vi "Main.vi"() -> ()   [LabVIEW 2020]
doc: "Main Program initialize config files, handles user inputs, image acquisition, object detection and image storing. User interface is handled in a state machine sending outputs."
uses:
  controls/State.ctl
  controls/Data.ctl
  <vilib>/userDefined/High Color/IMAQdx.ctl
  <vilib>/vision/Image Controls.llb/IMAQ Image.ctl
  b1a6e15a-21f6-4224-89c9-cebb1e441bce.vi
  4203ab90-da59-4329-829c-edbd02661f10.vi
  <extravilib>/ChannelInstances/Tag-bool/Read With Abort.vi
  <extravilib>/ChannelInstances/Tag-t'Data.ctl'/Read With Abort.vi
  <extravilib>/ChannelInstances/Tag-c(bool,bool)/Read With Abort.vi
  <extravilib>/ChannelInstances/Tag-c(bool,bool)/Write With Abort.vi
  <extravilib>/ChannelInstances/Tag-t'Data.ctl'/Write With Abort.vi
  <extravilib>/ChannelInstances/Tag-bool/Write With Abort.vi
  <extravilib>/ChannelInstances/Tag-c(bool,bool)/Instantiate.vi
  <extravilib>/ChannelInstances/Tag-t'Data.ctl'/Instantiate.vi
  <extravilib>/ChannelInstances/Tag-bool/Instantiate.vi
  <extravilib>/ChannelInstances/Tag-bool/EndpointRead.vi
  <extravilib>/ChannelInstances/Tag-t'Data.ctl'/EndpointRead.vi
  <extravilib>/ChannelInstances/Tag-c(bool,bool)/EndpointRead.vi
  <extravilib>/ChannelInstances/Tag-c(bool,bool)/Endpoint.vi
  <extravilib>/ChannelInstances/Tag-t'Data.ctl'/Endpoint.vi
  <extravilib>/ChannelInstances/Tag-bool/Endpoint.vi
  <extravilib>/ChannelInstances/Tag-bool.lvlib
  <extravilib>/ChannelInstances/Tag-t'Data.ctl'.lvlib
  <extravilib>/ChannelInstances/Tag-c(bool,bool).lvlib
panel:
  in  "Tab Control":T1(tab)
  in  "Sex":string="Station" caption="Sample Name"
  in  "Determiner":string="Station" caption="Sample Name"
  in  "Longitude":string="Station" caption="Sample Name"
  in  "Latitude":string="Station" caption="Sample Name"
  in  "Location":string="Station" caption="Sample Name"
  in  "Other notes":string caption="Sample Name"
  in  "Species Name":string="Test Sample" caption="Sample Name"
  in  "Station":string="Station" caption="Sample Name"
  in  "Collection date":string="24/06/2016" caption="Collection Date (DD/MM/YYYY)"
  out "Ready":bool
  in  "Operator":string="MRJ" caption="Sample Name"
  out "Active":bool
  in  "Start Image Capture":bool
  in  "Sample Name":string="#0000"
  in  "Stop Image Capture":bool
  out "Camera 2":bool
  out "Camear 1":bool
  out "Pump":bool
  out "Actuator":bool
  in  "Connect Systems":bool
  in  "Exit":bool
  in  "Empty and Refill":bool
  in  "Start System":bool
  in  "Empty System":bool
  out "Process buffer":T2(graph)
  out "Save buffer":T2(graph)
  in  "Close and Refill":bool
  in  "Manual Open":bool
  in  "Exposure Time":dbl=1000.0
  in  "Exposure":enum32{"Item 0", "Item 1", "Item 2", "Item 3"}(radio)=enum."Item 3"
  in  "Aperture":enum32{"Item 0", "Item 1", "Item 2", "Item 3"}(radio)
  in  "Flush Size":i32=100 min=0 max=1000
  in  "Dispense Duration":i32=200 min=20 max=200
  in  "Max large object threshold":i32=4 min=1
  in  "Change Crop":bool
  in  "DetectCrop":dbl=30.0 caption="Movement Detection size" format="%#_g %"
  in  "Sample size threshold":i32=500 min=1
  in  "New Sample timeout":i32=50 min=1
  out "Target framerate":i32=100
  in  "Light intensity":i32(slide)=100 min=1 max=100 scale=1.0..100.0 scale format="%.0f%"
  in  "Max Framerate":i32=100 min=1
  in  "Overload threshold":i32=50 min=1
  in  "Img Save Que Size":i32=100 caption="Image Save Queue Size" min=1
  in  "Img Proc Que Size":i32=200 caption="Image Processing Queue Size" min=1
  in  "Empty Cuvette":bool
  in  "Manual Close":bool
  out "Current Position":string
  in  "Position":bool
  in  "Pump Cycle":bool
  in  "Pump Bottom":bool
  in  "Pump Top":bool
  in  "Pump Terminate":bool
  in  "Override System":bool
  in  "Calibration Pictures":bool
  out "Framerate":i32 caption="Current Framerate"
  out "Camera 1":T3(plugin-control)
  out "Camera 2":T3(plugin-control)
  out "Camera 1 Binary":T3(plugin-control)
  out "Camera 2 Binary":T3(plugin-control)
  out "Camera 1 Detect":T3(plugin-control)
  out "Camera 2 Detect":T3(plugin-control)
  # "SRS Software - Version 1.5.3.2"
  # "Connections"
  # "Camera/Lens settings"
  # "Dispenser settings"
  # "Detection settings"
  # "Image capture settings"
  # "Buffer settings"
  # "Hatch control"
  # "Pump"
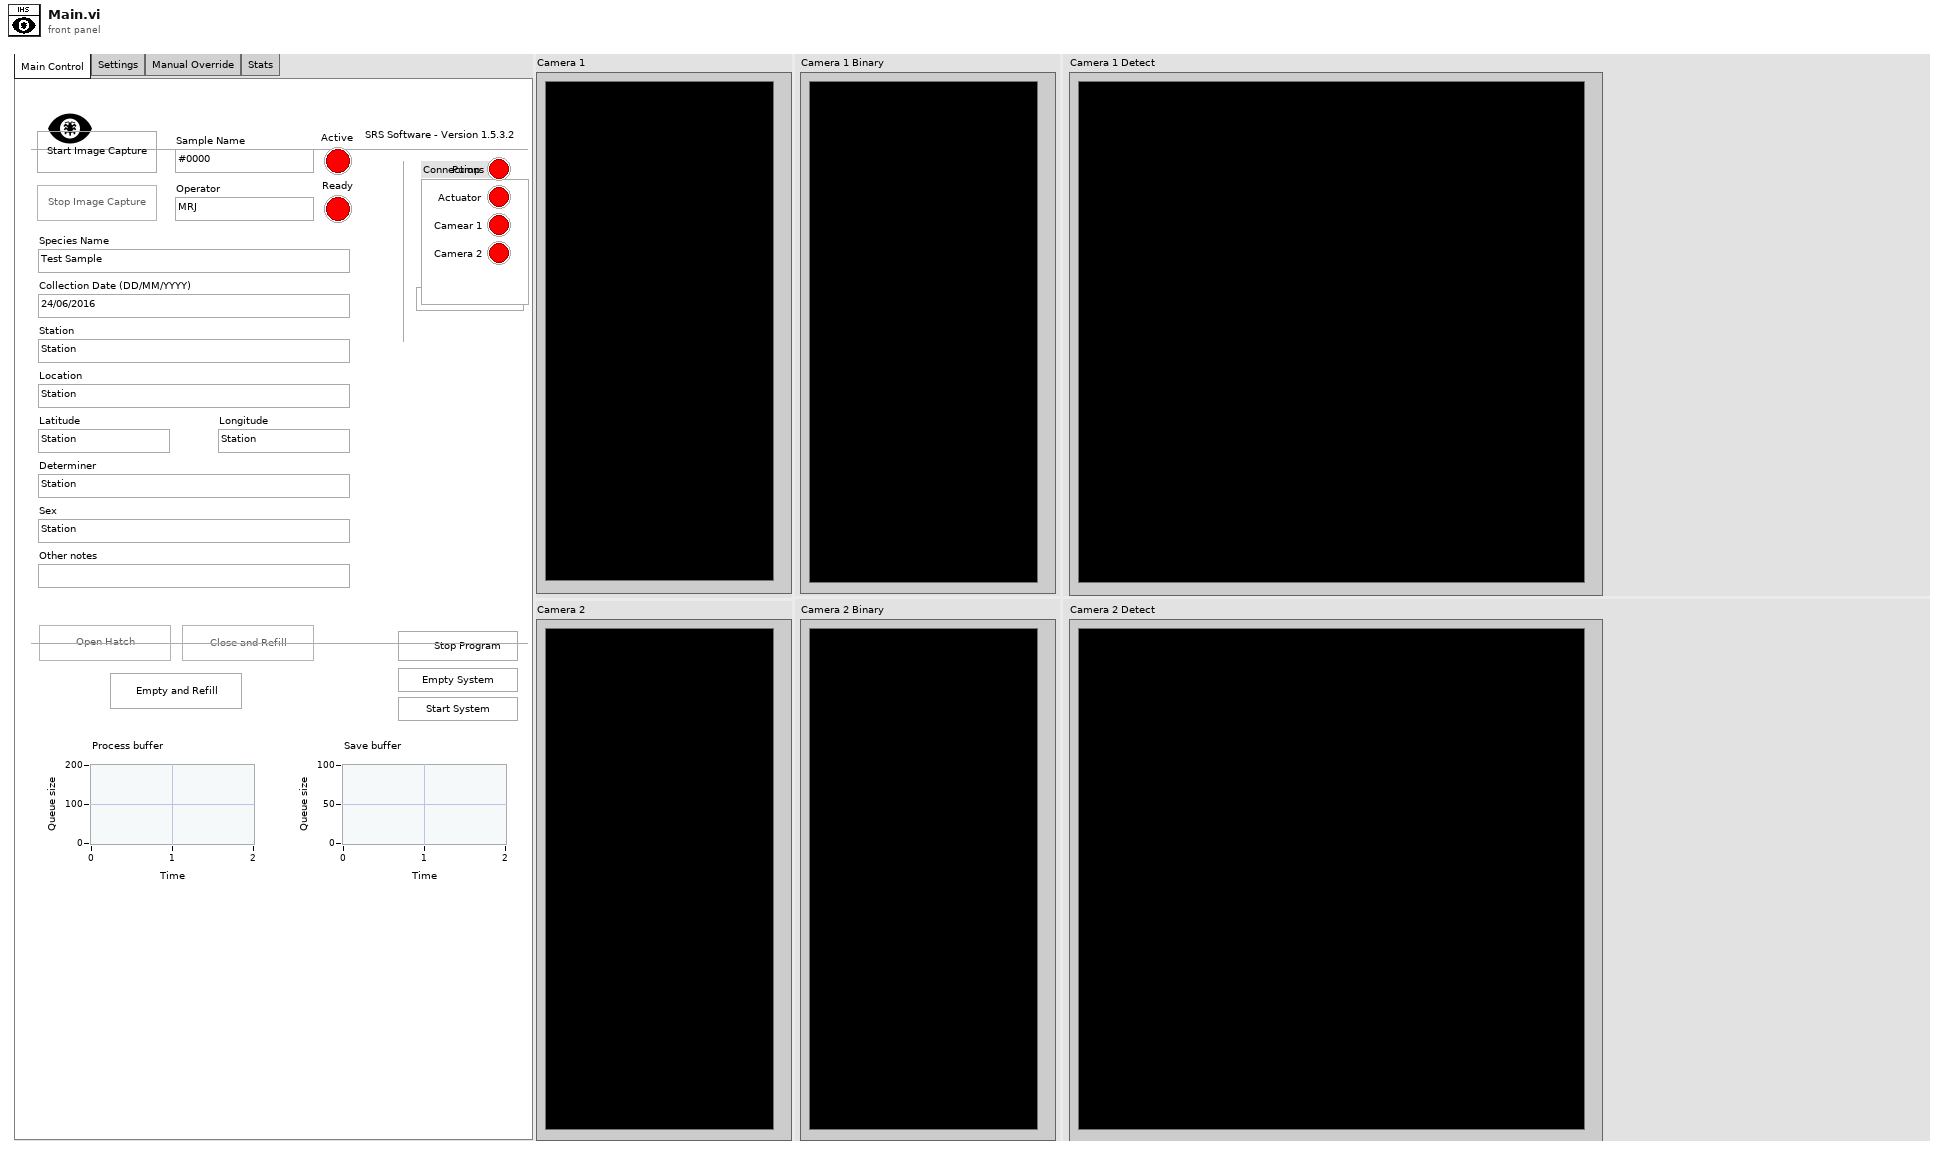
[diagram p1: front panel]
types:
  T1 = enum32{"Main Control", "Settings", "Manual Override", "Stats"}
  T2 = cluster{"# elements in queue":i32, "# elements in queue":i32}
  T3 = typedef "IMAQ Image.ctl" = refnum<image>
  T4 = typedef "Data.ctl" = cluster{"L16 Linear Actuator":refnum<visa-resource-name>, "XE 1000 Pump":refnum<visa-resource-name>, "Camera1":T5, "Camera2":T5, "Img_Capt":bool, "Actuator":bool, "Pump":bool, "Cam 1":bool, "Cam 2":bool, "Empty_Refill":bool, "Crop":bool, "Light intensity":i32, "Exposure Time":dbl, "Sample Name":string, "Operator":string, "Calibration 1":path, "Calibration 2":path, "Framerate":i32, "Timeout Sample":i32, "Collection date":string, "Sample size threshold":i32, "Empty start":u32, "Command":string, "Station":string, "Species Name":string, "Other Notes":string, "Aperture":enum32{"Item 0", "Item 1", "Item 2", "Item 3"}, "Image Process Queue Size":i32, "Image Save Queue Size":i32, "Overload threshold":i32, "Max Framerate":i32, "Rectangle 1":T6, "Rectangle 2":T6, "Detection Region %":dbl, "Detect 1":path, "Detect 2":path, "Max large object threshold":i32, "Open(T)/Close(F)":bool, "Img_Capt Begin":bool, "Dispense Speed":i32, "Flush Size":i32, "Location":string, "Latitude":string, "Longitude":string, "Determiner":string, "Sex":string, "Camera1_Img":T3, "Camera2_Img":T3, "Img1_Orig_Disp":T3, "Img2_Orig_Disp":T3, "Img1_Orig_RGB":T3, "Img2_Orig_RGB":T3, "Blue_Plane_Extract":T3, "Subtracted_Plane":T3, "Img1_Binary":T3, "Img2_Binary":T3, "Crop_Mask":T3, "Img1_Save":T3, "Img2_Save":T3, "Img1_Cali_Full":T3, "Img2_Cali_Full":T3, "Img1_Cali_Detect":T3, "Img2_Cali_Detect":T3, "Cam 1 queue":refnum<queue>, "Cam 1 - save queue":refnum<queue>, "Cam 2 queue":refnum<queue>, "Cam 2 - save queue":refnum<queue>}
  T5 = typedef "IMAQdx.ctl" = refnum<k21>
  T6 = typedef "IMAQ Rectangle" = cluster{"Left":i32, "Top":i32, "Right":i32, "Bottom":i32, "Rotation":dbl}
  T7 = typedef "State.ctl" = enum16{"Initialize", "Wait for Event", "Position", "Valve Signal", "Extra Flush", "Valve Cycle", "Valve Open", "Valve Close", "Pump Command", "Pump Cycle", "Empty System", "Start System", "Connect Systems", "Start Image Capture", "Stop Image Capture", "Calibration Pictures", "Close and Refill", "Empty and Refill", "Change Light Intensity", "Reconnect", "Exit"}
  T8 = enum8{"Enabled", "Disabled", "Disabled and Grayed Out"}
  T9 = cluster{"# elements in queue":i32, "# elements in queue":i32}[]
  T10 = typedef "Tag-t'Data.ctl'.lvlib/))Channel.ctl" = refnum<queue>
  T11 = typedef "Tag-bool.lvlib/))Channel.ctl" = refnum<queue>
  T12 = typedef "Tag-c(bool,bool).lvlib/))Channel.ctl" = refnum<queue>
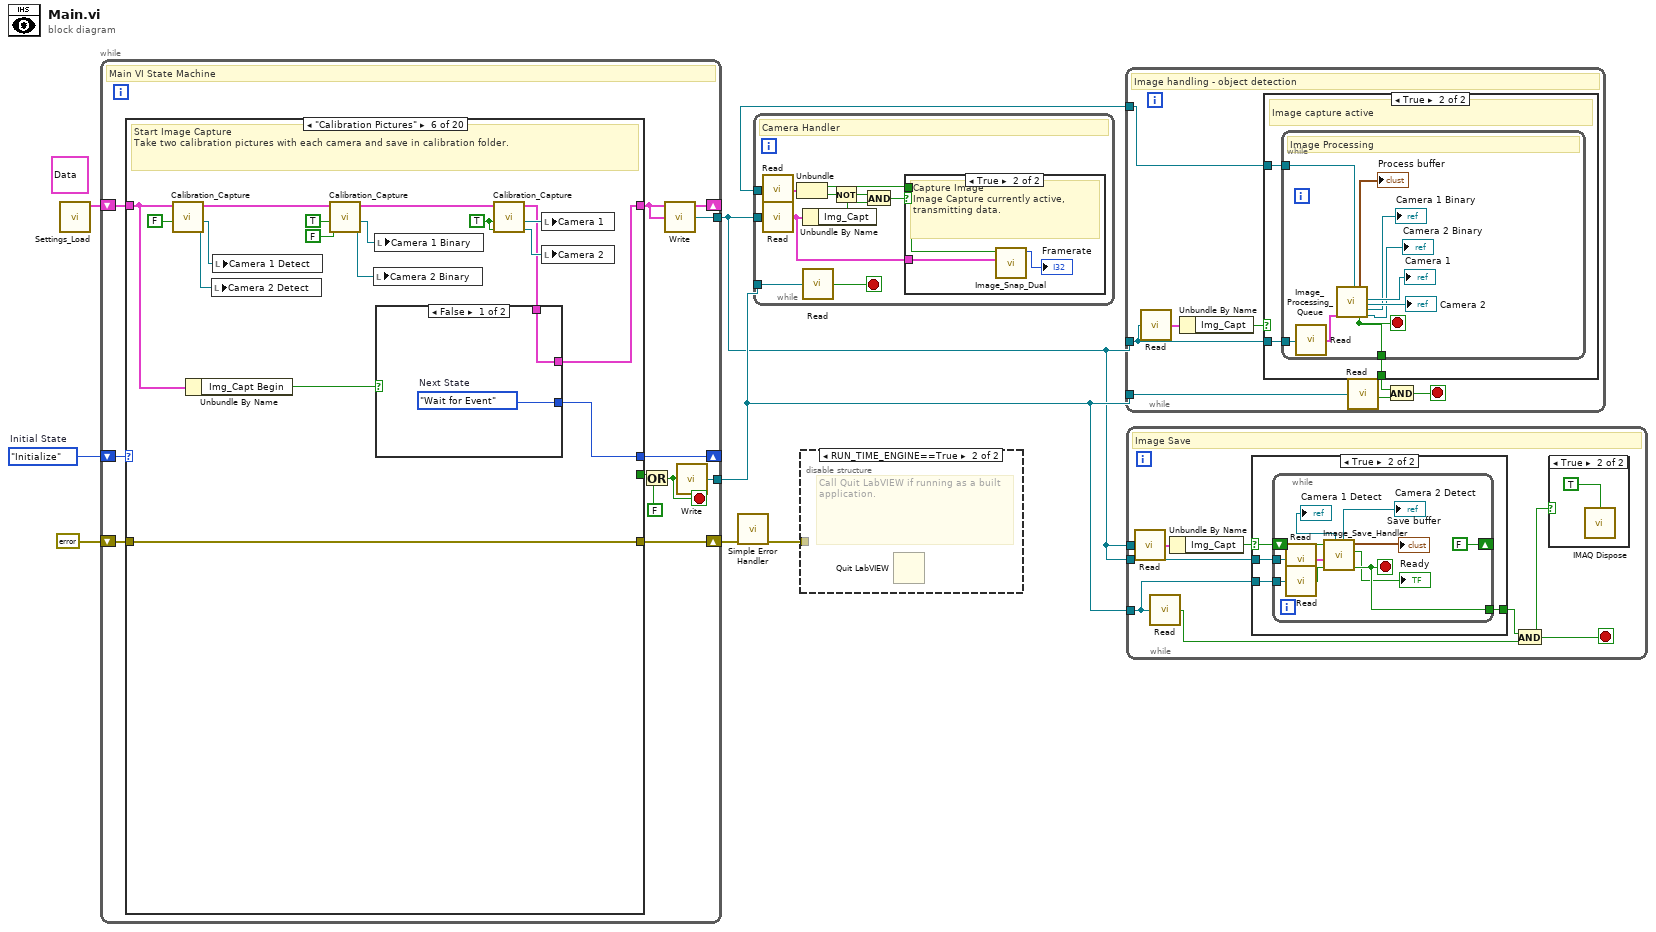
[diagram p0: block diagram]
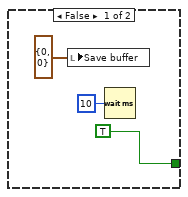
[diagram p3: hidden frame]
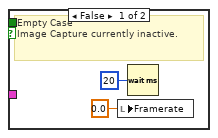
[diagram p4: hidden frame]
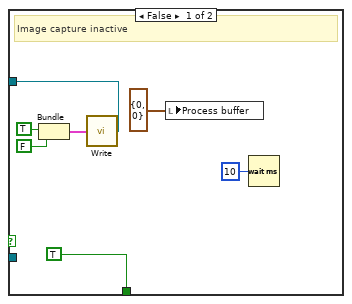
[diagram p5: hidden frame]
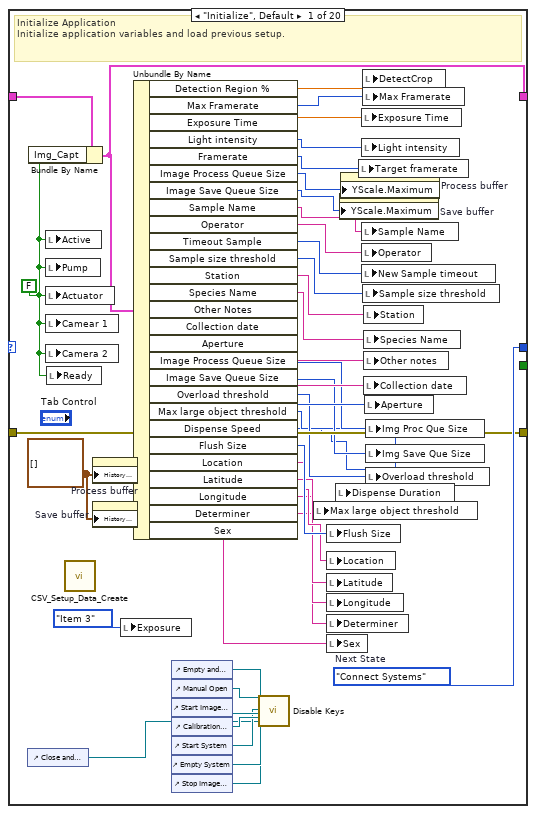
[diagram p7: hidden frame]
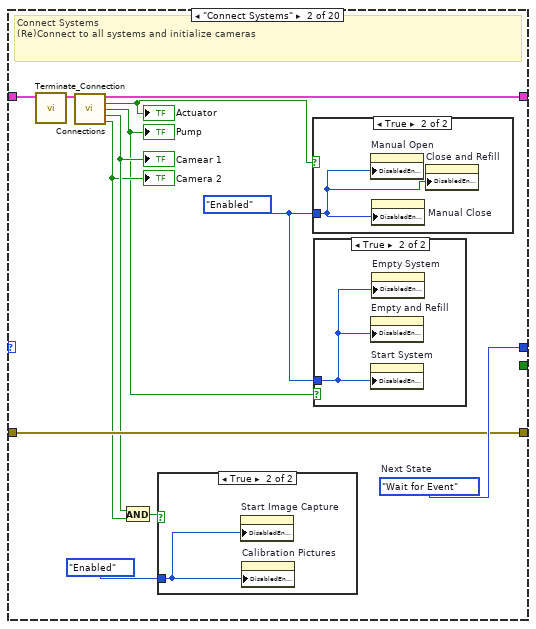
[diagram p8: hidden frame]
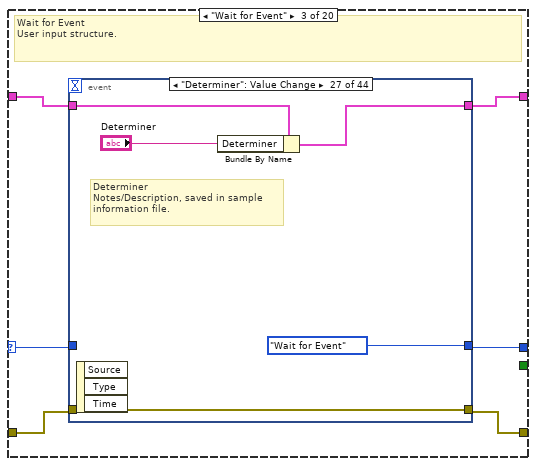
[diagram p12: hidden frame]
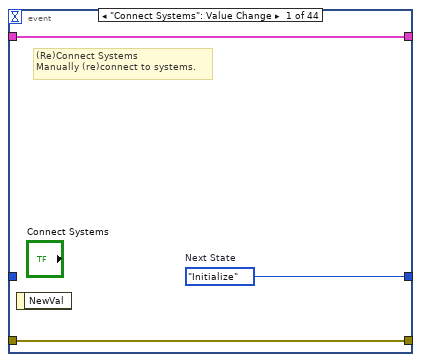
[diagram p13: hidden frame]
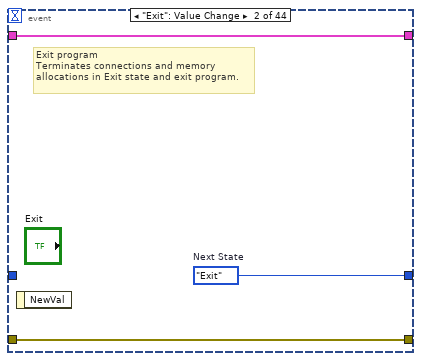
[diagram p14: hidden frame]
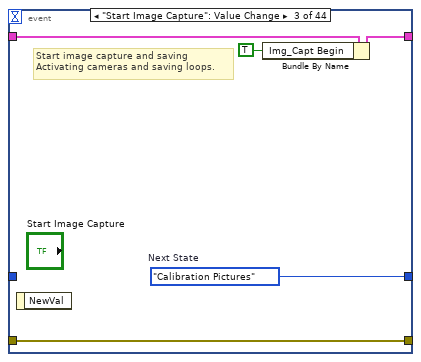
[diagram p15: hidden frame]
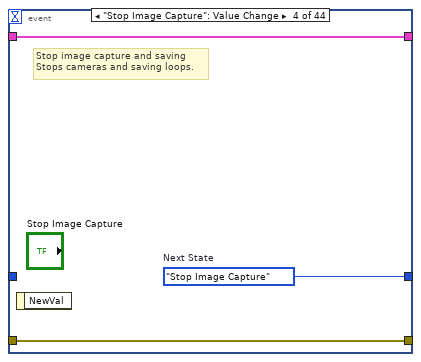
[diagram p16: hidden frame]
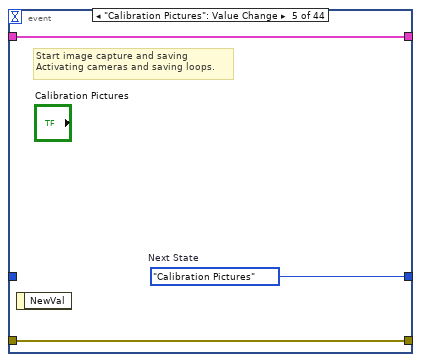
[diagram p17: hidden frame]
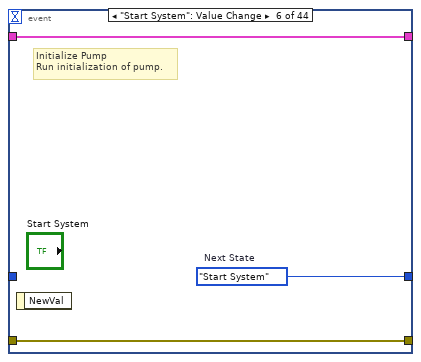
[diagram p18: hidden frame]
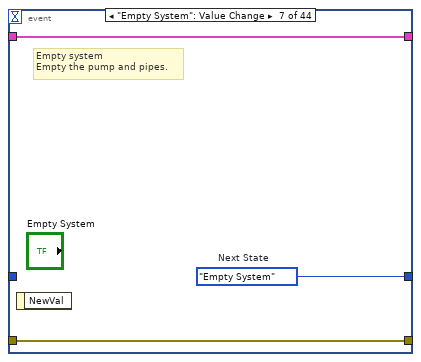
[diagram p19: hidden frame]
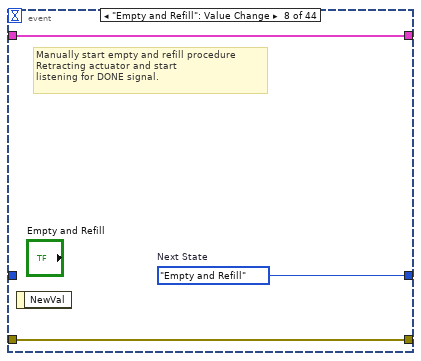
[diagram p20: hidden frame]
diagram:
  (unwired) T4 {"L16 Linear Actuator"="", "XE 1000 Pump"="", "Camera1"="", "Camera2"="", "Img_Capt"=FALSE, "Actuator"=FALSE, "Pump"=FALSE, "Cam 1"=FALSE, "Cam 2"=FALSE, "Empty_Refill"=FALSE, "Crop"=FALSE, "Light intensity"=100, "Exposure Time"=1000.0, "Sample Name"="Test Sample", "Operator"="MRJ", "Calibration 1"=path "C:/Users/au540322/Desktop/IHS_Project/images/Debris/Debris_0/Debris_0_2019_06_01-23-32-49-686.PNG", "Calibration 2"=path "C:/Users/au540322/Desktop/IHS_Project/images/Debris/Debris_0/Debris_0_2019_06_01-23-32-49-686.PNG", "Framerate"=100, "Timeout Sample"=200, "Collection date"="", "Sample size threshold"=500, "Empty start"=1, "Command"="", "Station"="", "Species Name"="", "Other Notes"="", "Aperture"=enum."Item 0", "Image Process Queue Size"=500, "Image Save Queue Size"=500, "Overload threshold"=500, "Max Framerate"=100, "Rectangle 1"={"Left"=0, "Top"=0, "Right"=0, "Bottom"=0, "Rotation"=0.0}, "Rectangle 2"={"Left"=0, "Top"=0, "Right"=0, "Bottom"=0, "Rotation"=0.0}, "Detection Region %"=0.0, "Detect 1"=path "C:/Users/au540322/Desktop/IHS_Project/images/Debris/Debris_0/Debris_0_2019_06_01-23-32-49-686.PNG", "Detect 2"=path "C:/Users/au540322/Desktop/IHS_Project/images/Debris/Debris_0/Debris_0_2019_06_01-23-32-49-686.PNG", "Max large object threshold"=0, "Open(T)/Close(F)"=FALSE, "Img_Capt Begin"=FALSE, "Dispense Speed"=100, "Flush Size"=100, "Location"="Station", "Latitude"="Station", "Longitude"="Station", "Determiner"="Station", "Sex"="Station", "Camera1_Img"=refnum, "Camera2_Img"=refnum, "Img1_Orig_Disp"=refnum, "Img2_Orig_Disp"=refnum, "Img1_Orig_RGB"=refnum, "Img2_Orig_RGB"=refnum, "Blue_Plane_Extract"=refnum, "Subtracted_Plane"=refnum, "Img1_Binary"=refnum, "Img2_Binary"=refnum, "Crop_Mask"=refnum, "Img1_Save"=refnum, "Img2_Save"=refnum, "Img1_Cali_Full"=refnum, "Img2_Cali_Full"=refnum, "Img1_Cali_Detect"=refnum, "Img2_Cali_Detect"=refnum, "Cam 1 queue"=refnum, "Cam 1 - save queue"=refnum, "Cam 2 queue"=refnum, "Cam 2 - save queue"=refnum} ("Data")
  w8 = State."Initialize"  # Initial State
  n1 = call "Settings_Load.vi"() -> ("value"=w4:T4)  [unwired: 10 in, 1 out]
  n2 = while {
    shift-right: [w18] -> _
    shift-left: w8 -> [w19]
    shift-right: [w16] -> _
    shift-left: w4 -> [w17]
    shift-right: [w13] -> w6
    shift-left: errorcluster {"status"=FALSE, "code"=0, "source"=""} ("error constant") -> [w15]
    tunnel: [w10] -> w3
    tunnel: [w11] -> w2
    stop <- w14 stop-if-true
    # "Main VI State Machine"
    n3 = case shown="\"Calibration Pictures\"" w19 {
      selector: w19 -> [_ _ w77 _ _ _ _ _ _ _ _ _ _ _ _ _ _ _ _ _]
      tunnel: [w61 w73 w82 w311 w329 w347 w376 w401 w407 w424 w441 w449 w462 w480 w490 w520 w542 w560 w563 w576] -> w18
      tunnel: [_ _ _ _ _ _ _ _ _ _ _ _ _ _ _ _ _ _ _ w575] -> w12
      tunnel: w17 -> [w53 w70 w81 w312 w325 w340 w370 w395 w411 w428 w433 w447 w460 w479 w484 w519 w532 w544 w567 w569]
      tunnel: [w59 w71 w80 w313 w327 w339 w375 w400 w402 w428 w434 w444 w459 w479 w483 w519 w531 w543 w567 w572] -> w16
      tunnel: w15 -> [w60 w72 w79 w314 w328 w346 w365 w390 w410 w425 w439 w452 w464 w475 w487 w516 w539 w557 w566 w574]
      tunnel: [w60 w72 w78 w314 w328 w346 w359 w383 w410 w418 w438 w450 w453 w474 w486 w513 w538 w548 w564 w568] -> w13
      frame "Initialize", Default {
        w52 = T9 [] ("History Data")
        w51 = FALSE ("Pump")
        w61 = State."Connect Systems"  # Next State
        # "Initialize Application\nInitialize application variables and load previous setup."
        n4 = control-ref of="Close and Refill"() -> (w33:refnum<vi>)
        n5 = Bundle By Name(cluster=w53, "Img_Capt"=w51) -> (w59:T4)
        n6 = local write "Active"(w51) -> ()
        n7 = local write "Pump"(w51) -> ()
        n8 = local write "Actuator"(w51) -> ()
        n9 = local write "Camear 1"(w51) -> ()
        n10 = local write "Camera 2"(w51) -> ()
        n11 = local write "Ready"(w51) -> ()
        n12 = call "CSV_Setup_Data_Create.vi"() -> ()  [unwired: 11 in, 1 out]
        n13 = property on="Process buffer" class="WFChart (strict)"("History Data"=w52) -> ()  [unwired: 2 in, 2 out]
        n14 = property on="Save buffer" class="WFChart (strict)"("History Data"=w52) -> ()  [unwired: 2 in, 2 out]
        n15 = local write "Exposure"(enum32{"Item 0", "Item 1", "Item 2", "Item 3"}."Item 3" ("Exposure")) -> ()
        n16 = Unbundle By Name(w59) -> ("Detection Region %"=w30:dbl, "Max Framerate"=w31:i32, "Exposure Time"=w58:dbl, "Light intensity"=w57:i32, "Framerate"=w56:i32, "Image Process Queue Size"=w29:i32, "Image Save Queue Size"=w28:i32, "Sample Name"=w55:string, "Operator"=w54:string, "Timeout Sample"=w50:i32, "Sample size threshold"=w49:i32, "Station"=w48:string, "Species Name"=w47:string, "Other Notes"=w46:string, "Collection date"=w45:string, "Aperture"=w44:enum32{"Item 0", "Item 1", "Item 2", "Item 3"}, "Image Process Queue Size"=w43:i32, "Image Save Queue Size"=w42:i32, "Overload threshold"=w41:i32, "Max large object threshold"=w27:i32, "Dispense Speed"=w25:i32, "Flush Size"=w26:i32, "Location"=w24:string, "Latitude"=w23:string, "Longitude"=w22:string, "Determiner"=w21:string, "Sex"=w20:string)
        n17 = control-ref of="Empty and Refill"() -> (w40:refnum<vi>)
        n18 = control-ref of="Manual Open"() -> (w39:refnum<vi>)
        n19 = control-ref of="Start Image Capture"() -> (w37:refnum<vi>)
        n20 = control-ref of="Calibration Pictures"() -> (w38:refnum<vi>)
        n21 = control-ref of="Start System"() -> (w36:refnum<vi>)
        n22 = control-ref of="Empty System"() -> (w35:refnum<vi>)
        n23 = control-ref of="Stop Image Capture"() -> (w34:refnum<vi>)
        n24 = call "Disable Keys.vi"("Boolean in"=w39, "Bool Refnum 6"=w40, "Bool Refnum 4"=w34, "Bool Refnum 7"=w36, "Bool Refnum 9"=w37, "Bool Refnum 2"=w38, "Bool Refnum 8"=w33, "Bool Refnum 3"=w35) -> ()  [unwired: 20 in]
        n25 = local write "Max large object threshold"(w27) -> ()
        n26 = local write "Flush Size"(w26) -> ()
        n27 = local write "Location"(w24) -> ()
        n28 = local write "Latitude"(w23) -> ()
        n29 = local write "Longitude"(w22) -> ()
        n30 = local write "Determiner"(w21) -> ()
        n31 = local write "Sex"(w20) -> ()
        n32 = local write "Dispense Duration"(w25) -> ()
        n33 = property on="Save buffer" class="WFChart (strict)"("YScale.Maximum"=w28) -> ()  [unwired: 2 in, 2 out]
        n34 = property on="Process buffer" class="WFChart (strict)"("YScale.Maximum"=w29) -> ()  [unwired: 2 in, 2 out]
        n35 = local write "Target framerate"(w56) -> ()
        n36 = local write "Exposure Time"(w58) -> ()
        n37 = local write "Light intensity"(w57) -> ()
        n38 = local write "Sample Name"(w55) -> ()
        n39 = local write "Operator"(w54) -> ()
        n40 = local write "New Sample timeout"(w50) -> ()
        n41 = local write "DetectCrop"(w30) -> ()
        n42 = local write "Max Framerate"(w31) -> ()
        n43 = local write "Sample size threshold"(w49) -> ()
        n44 = local write "Station"(w48) -> ()
        n45 = local write "Species Name"(w47) -> ()
        n46 = local write "Other notes"(w46) -> ()
        n47 = local write "Collection date"(w45) -> ()
        n48 = local write "Aperture"(w44) -> ()
        n49 = local write "Img Proc Que Size"(w43) -> ()
        n50 = local write "Img Save Que Size"(w42) -> ()
        n51 = local write "Overload threshold"(w41) -> ()
      }
      frame "Connect Systems" {
        w62 = T8."Enabled" ("Disabled")
        w73 = State."Wait for Event"  # Next State
        # "Connect Systems\n(Re)Connect to all systems and initialize cameras"
        n52 = call "Terminate_Connection.vi"("Data"=w70) -> ("Data out"=w69:T4)  [unwired: 9 in, 1 out]
        n53 = call "Connections.vi"("input cluster"=w69) -> ("output cluster"=w71:T4, "Linear Actuator"=w68:bool, "Pump"=w64:bool, "Camear 1"=w66:bool, "Camera 2"=w65:bool)  [unwired: 10 in]
        "Pump" <- w64
        "Actuator" <- w68
        "Camera 2" <- w65
        "Camear 1" <- w66
        n54 = And(x=w66, y=w65) -> (x .and. y?=w67:bool)
        n55 = case shown="True" w67 {
          tunnel: T8."Enabled" ("Disabled") -> [_ w75]
          frame False {
          }
          frame True {
            n56 = property on="Start Image Capture" class="Bool"("DisabledEnum"=w75) -> ()  [unwired: 2 in, 2 out]
            n57 = property on="Calibration Pictures" class="Bool"("DisabledEnum"=w75) -> ()  [unwired: 2 in, 2 out]
          }
        }
        n58 = case shown="True" w68 {
          tunnel: w62 -> [_ w76]
          frame False {
          }
          frame True {
            n59 = property on="Manual Open" class="Bool"("DisabledEnum"=w76) -> ()  [unwired: 2 in, 2 out]
            n60 = property on="Manual Close" class="Bool"("DisabledEnum"=w76) -> ()  [unwired: 2 in, 2 out]
            n61 = property on="Close and Refill" class="Bool"("DisabledEnum"=w76) -> ()  [unwired: 2 in, 2 out]
          }
        }
        n62 = case shown="True" w64 {
          tunnel: w62 -> [_ w74]
          frame False {
          }
          frame True {
            n63 = property on="Empty and Refill" class="Bool"("DisabledEnum"=w74) -> ()  [unwired: 2 in, 2 out]
            n64 = property on="Start System" class="Bool"("DisabledEnum"=w74) -> ()  [unwired: 2 in, 2 out]
            n65 = property on="Empty System" class="Bool"("DisabledEnum"=w74) -> ()  [unwired: 2 in, 2 out]
          }
        }
      }
      frame "Wait for Event" {
        # "Wait for Event\nUser input structure."
        n66 = event shown="[26] \"Determiner\": Value Change" {
          selector: _ -> [_ _ _ _ _ _ _ _ _ _ _ _ _ _ _ _ _ _ _ _ _ _ _ _ _ _ _ _ _ _ _ _ _ _ _ _ _ _ _ _ _ _ _ _]
          dyn-events: _ -> [_ _ _ _ _ _ _ _ _ _ _ _ _ _ _ _ _ _ _ _ _ _ _ _ _ _ _ _ _ _ _ _ _ _ _ _ _ _ _ _ _ _ _ _]
          timeout: _ -> [_ _ _ _ _ _ _ _ _ _ _ _ _ _ _ _ _ _ _ _ _ _ _ _ _ _ _ _ _ _ _ _ _ _ _ _ _ _ _ _ _ _ _ _]
          tunnel: [w85 w88 w93 w96 w99 w102 w105 w108 w111 w122 w125 w128 w131 w134 w137 w142 w147 w152 w153 w158 State."Wait for Event" ("Next State") State."Wait for Event" ("Next State") State."Wait for Event" ("Next State") State."Wait for Event" ("Next State") State."Wait for Event" ("Next State") State."Wait for Event" ("Next State") State."Wait for Event" ("Next State") State."Wait for Event" ("Next State") State."Wait for Event" ("Next State") State."Wait for Event" ("Next State") State."Wait for Event" ("Next State") State."Wait for Event" ("Next State") w245 w250 w255 w260 w265 w277 State."Change Light Intensity" ("Next State") w286 w291 State."Change Light Intensity" ("Next State") State."Wait for Event" ("Next State") w308] -> w82
          tunnel: w81 -> [w83 w87 w91 w94 w97 w100 w103 w106 w109 w120 w123 w126 w129 w132 w135 w139 w144 w149 w156 w159 w164 w168 w174 w179 w184 w189 w194 w199 w204 w211 w216 w239 w246 w251 w256 w261 w266 w270 w283 w288 w293 w298 w303 w306]
          tunnel: [w83 w87 w90 w94 w97 w100 w103 w106 w109 w120 w123 w126 w129 w132 w135 w138 w143 w148 w155 w160 w165 w169 w175 w180 w185 w190 w195 w200 w205 w208 w224 w240 w247 w252 w257 w262 w267 w278 w282 w287 w292 w297 w302 w305] -> w80
          tunnel: w79 -> [w84 w86 w92 w95 w98 w101 w104 w107 w110 w121 w124 w127 w130 w133 w136 w141 w146 w151 w157 w162 w167 w172 w177 w182 w187 w192 w197 w202 w207 w213 w226 w243 w248 w253 w258 w263 w268 w279 w284 w289 w294 w299 w304 w307]
          tunnel: [w84 w86 w92 w95 w98 w101 w104 w107 w110 w121 w124 w127 w130 w133 w136 w141 w146 w151 w157 w162 w167 w172 w177 w182 w187 w192 w197 w202 w207 w213 w226 w243 w248 w253 w258 w263 w268 w279 w284 w289 w294 w299 w304 w307] -> w78
          tunnel: w77 -> [_ _ _ _ _ _ _ _ _ _ _ _ _ _ _ _ _ _ _ _ _ _ _ _ _ _ _ _ _ _ _ _ _ _ _ _ _ _ _ _ _ _ _ _]
          event "Connect Systems": Value Change {
            w85 = State."Initialize"  # Next State
            # "(Re)Connect Systems\nManually (re)connect to systems."
            n67 = event-data() -> ()  [unwired: 1 in, 1 out]
          }
          event "Exit": Value Change {
            w88 = State."Exit"  # Next State
            # "Exit program\nTerminates connections and memory\nallocations in Exit state and exit program."
            n68 = event-data() -> ()  [unwired: 1 in, 1 out]
          }
          event "Start Image Capture": Value Change {
            w93 = State."Calibration Pictures"  # Next State
            # "Start image capture and saving\nActivating cameras and saving loops."
            n69 = event-data() -> ()  [unwired: 1 in, 1 out]
            n70 = Bundle By Name(cluster=w91, "Img_Capt Begin"=TRUE) -> (w90:T4)
          }
          event "Stop Image Capture": Value Change {
            w96 = State."Stop Image Capture"  # Next State
            # "Stop image capture and saving\nStops cameras and saving loops."
            n71 = event-data() -> ()  [unwired: 1 in, 1 out]
          }
          event "Calibration Pictures": Value Change {
            w99 = State."Calibration Pictures"  # Next State
            # "Start image capture and saving\nActivating cameras and saving loops."
            n72 = event-data() -> ()  [unwired: 1 in, 1 out]
          }
          event "Start System": Value Change {
            w102 = State."Start System"  # Next State
            # "Initialize Pump\nRun initialization of pump."
            n73 = event-data() -> ()  [unwired: 1 in, 1 out]
          }
          event "Empty System": Value Change {
            w105 = State."Empty System"  # Next State
            # "Empty system\nEmpty the pump and pipes."
            n74 = event-data() -> ()  [unwired: 1 in, 1 out]
          }
          event "Empty and Refill": Value Change {
            w108 = State."Empty and Refill"  # Next State
            # "Manually start empty and refill procedure\nRetracting actuator and start \nlistening for DONE signal."
            n75 = event-data() -> ()  [unwired: 1 in, 1 out]
          }
          event "Close and Refill": Value Change {
            w111 = State."Close and Refill"  # Next State
            # "Manually start empty and refill procedure\nRetracting actuator and start \nlistening for DONE signal."
            n76 = event-data() -> ()  [unwired: 1 in, 1 out]
          }
          event "Override System": Value Change {
            w122 = State."Wait for Event"  # Next State
            # "Override System\nAllowing full access to systems"
            n77 = event-data() -> ()  [unwired: 1 in, 1 out]
            n78 = control-ref of="Empty and Refill"() -> (w112:refnum<vi>)
            n79 = control-ref of="Start Image Capture"() -> (w113:refnum<vi>)
            n80 = control-ref of="Manual Open"() -> (w114:refnum<vi>)
            n81 = control-ref of="Manual Open"() -> (w115:refnum<vi>)
            n82 = control-ref of="Calibration Pictures"() -> (w116:refnum<vi>)
            n83 = control-ref of="Empty System"() -> (w117:refnum<vi>)
            n84 = control-ref of="Start System"() -> (w118:refnum<vi>)
            n85 = control-ref of="Stop Image Capture"() -> (w119:refnum<vi>)
            n86 = call "Enable Keys.vi"("Boolean in"=w112, "Bool Refnum 2"=w113, "Bool Refnum 3"=w114, "Bool Refnum 4"=w115, "Bool Refnum 6"=w116, "Bool Refnum 7"=w117, "Bool Refnum 8"=w118, "Bool Refnum 9"=w119) -> ()  [unwired: 20 in]
          }
          event "Empty Cuvette": Value Change {
            w125 = State."Valve Cycle"  # Next State
            # "Manual cycle of linear actuator\nRetract and extends linear actuator."
            n87 = event-data() -> ()  [unwired: 1 in, 1 out]
          }
          event "Manual Open": Value Change {
            w128 = State."Valve Open"  # Next State
            # "Manual extend\nManually extend linear actuator."
            n88 = event-data() -> ()  [unwired: 1 in, 1 out]
          }
          event "Manual Close": Value Change {
            w131 = State."Valve Close"  # Next State
            # "Manual Retract\nManually retract linear actuator."
            n89 = event-data() -> ()  [unwired: 1 in, 1 out]
          }
          event "Position": Value Change {
            w134 = State."Position"  # Next State
            # "Read position\nRead linear actuator position."
            n90 = event-data() -> ()  [unwired: 1 in, 1 out]
          }
          event "Pump Cycle": Value Change {
            w137 = State."Pump Cycle"  # Next State
            # "Manual Pump Cycle\nManually go through a pump cycle."
            n91 = event-data() -> ()  [unwired: 1 in, 1 out]
          }
          event "Pump Top": Value Change {
            w142 = State."Pump Command"  # Next State
            # "Manual Move Pump Top\nManually move the pump \nto the top position."
            n92 = event-data() -> ()  [unwired: 1 in, 1 out]
            n93 = Bundle By Name(cluster=w139, "Command"="A1000R" ("write buffer 2")) -> (w138:T4)
          }
          event "Pump Bottom": Value Change {
            w147 = State."Pump Command"  # Next State
            # "Manual Move Pump Bottom\nManually move the pump\nto the bottom position."
            n94 = event-data() -> ()  [unwired: 1 in, 1 out]
            n95 = Bundle By Name(cluster=w144, "Command"="A0R" ("write buffer 2")) -> (w143:T4)
          }
          event "Pump Terminate": Value Change {
            w152 = State."Pump Command"  # Next State
            # "Terminate Pump\nAbort all current pump commands, \nacts as emergency stop."
            n96 = event-data() -> ()  [unwired: 1 in, 1 out]
            n97 = Bundle By Name(cluster=w149, "Command"="T" ("write buffer 2")) -> (w148:T4)
          }
          event "Sample Name": Value Change {
            w153 = State."Wait for Event"  # Next State
            # "Sample Name\nSample Name, used in image folders,\nand saved in sample information file."
            n98 = event-data() -> ()  [unwired: 1 in, 3 out]
            n99 = Bundle By Name(cluster=w156, "Sample Name"="Sample Name") -> (w155:T4)
          }
          event "Operator": Value Change {
            w158 = State."Wait for Event"  # Next State
            # "Operator Name\nOperator Name, saved in sample information file."
            n100 = event-data() -> ()  [unwired: 1 in, 3 out]
            n101 = Bundle By Name(cluster=w159, "Operator"="Operator") -> (w160:T4)
          }
          event "Species Name": Value Change {
            # "Sample Notes\nNotes/Description, saved in sample \ninformation file."
            n102 = event-data() -> ()  [unwired: 1 in, 3 out]
            n103 = Bundle By Name(cluster=w164, "Species Name"="Species Name") -> (w165:T4)
          }
          event "Collection date": Value Change {
            # "Sample Notes\nNotes/Description, saved in sample \ninformation file."
            n104 = event-data() -> ()  [unwired: 1 in, 3 out]
            n105 = Bundle By Name(cluster=w168, "Collection date"="Collection date") -> (w169:T4)
          }
          event "Station": Value Change {
            # "Sample Notes\nNotes/Description, saved in sample \ninformation file."
            n106 = event-data() -> ()  [unwired: 1 in, 3 out]
            n107 = Bundle By Name(cluster=w174, "Station"="Station") -> (w175:T4)
          }
          event "Location": Value Change {
            # "Location\nNotes/Description, saved in sample \ninformation file."
            n108 = event-data() -> ()  [unwired: 1 in, 3 out]
            n109 = Bundle By Name(cluster=w179, "Location"="Location") -> (w180:T4)
          }
          event "Latitude": Value Change {
            # "Latitude\nNotes/Description, saved in sample \ninformation file."
            n110 = event-data() -> ()  [unwired: 1 in, 3 out]
            n111 = Bundle By Name(cluster=w184, "Latitude"="Latitude") -> (w185:T4)
          }
          event "Longitude": Value Change {
            # "Longitude\nNotes/Description, saved in sample \ninformation file."
            n112 = event-data() -> ()  [unwired: 1 in, 3 out]
            n113 = Bundle By Name(cluster=w189, "Longitude"="Longitude") -> (w190:T4)
          }
          event "Determiner": Value Change {
            # "Determiner\nNotes/Description, saved in sample \ninformation file."
            n114 = event-data() -> ()  [unwired: 1 in, 3 out]
            n115 = Bundle By Name(cluster=w194, "Determiner"="Determiner") -> (w195:T4)
          }
          event "Sex": Value Change {
            # "Sex\nNotes/Description, saved in sample \ninformation file."
            n116 = event-data() -> ()  [unwired: 1 in, 3 out]
            n117 = Bundle By Name(cluster=w199, "Sex"="Sex") -> (w200:T4)
          }
          event "Other notes": Value Change {
            # "Sample Notes\nNotes/Description, saved in sample \ninformation file."
            n118 = event-data() -> ()  [unwired: 1 in, 3 out]
            n119 = Bundle By Name(cluster=w204, "Other Notes"="Other notes") -> (w205:T4)
          }
          event "Aperture": Value Change {
            # "Aperture\nAperture setting (manually changed on cameras)\nsaved in information file. Loads calibration image."
            n120 = event-data() -> ()  [unwired: 1 in, 3 out]
            n121 = Bundle By Name(cluster=w211, "Aperture"="Aperture") -> (w209:T4)
            n122 = call "Calibration_Update.vi"("value"=w209) -> ("output cluster"=w208:T4)  [unwired: 10 in]
          }
          event "Exposure": Value Change {
            n123 = event-data() -> ()  [unwired: 1 in, 3 out]
            n124 = Unbundle By Name(w216) -> ("Max Framerate"=w221:i32)
            n125 = case shown="\"Item 3\"" "Exposure" {
              tunnel: [1000.0 1500.0 2000.0 w230] -> w214
              frame "Item 0", Default {
              }
              frame "Item 1" {
              }
              frame "Item 2" {
              }
              frame "Item 3" {
                n126 = local read "Exposure Time"() -> (w230:dbl)
              }
            }
            n127 = Multiply(x=w214, y=10.0) -> (x*y=w219:dbl)
            n128 = Divide(x=1000000.0, y=w219) -> (x/y=w220:dbl)
            n129 = Max & Min(x=w220, y=w221) -> (min(x,y)=w222:dbl)  [unwired: 1 out]
            n130 = local write "Exposure Time"(w214) -> ()
            n131 = Bundle By Name(cluster=w216, "Exposure Time"=w214, "Framerate"=w222) -> (w215:T4)
            n132 = local write "Target framerate"(w222) -> ()
            n133 = call "Calibration_Update.vi"("value"=w215) -> ("output cluster"=w224:T4)  [unwired: 10 in]
          }
          event "Exposure Time": Value Change {
            # "Exposure Time\nChanges camera exposure time, must restart image\nacquisition to enable new value. Value is saved in \nsample information file."
            n134 = event-data() -> ()  [unwired: 1 in, 3 out]
            n135 = Unbundle By Name(w239) -> ("Max Framerate"=w233:i32)
            n136 = Multiply(x="Exposure Time", y=10.0) -> (x*y=w236:dbl)
            n137 = Divide(x=1000000.0, y=w236) -> (x/y=w234:dbl)
            n138 = Max & Min(x=w234, y=w233) -> (min(x,y)=w232:dbl)  [unwired: 1 out]
            "Target framerate" <- w232
            n139 = Bundle By Name(cluster=w239, "Exposure Time"="Exposure Time", "Framerate"=w232) -> (w241:T4)
            n140 = local write "Exposure"(enum32{"Item 0", "Item 1", "Item 2", "Item 3"}."Item 3" ("Exposure")) -> ()
            n141 = call "Calibration_Update.vi"("value"=w241) -> ("output cluster"=w240:T4)  [unwired: 10 in]
          }
          event "Img Proc Que Size": Value Change {
            w245 = State."Wait for Event"  # Next State
            # "Image Processing Queue Size\nMaximum buffer size of the image processing queue."
            n142 = event-data() -> ()  [unwired: 1 in, 3 out]
            n143 = Bundle By Name(cluster=w246, "Image Process Queue Size"="Img Proc Que Size") -> (w247:T4)
            n144 = property on="Process buffer" class="WFChart (strict)"("YScale.Maximum"="Img Proc Que Size") -> ()  [unwired: 2 in, 2 out]
          }
          event "Img Save Que Size": Value Change {
            w250 = State."Wait for Event"  # Next State
            # "Image Save Queue Size\nMaximum buffer size of the image saving queue."
            n145 = event-data() -> ()  [unwired: 1 in, 3 out]
            n146 = Bundle By Name(cluster=w251, "Image Save Queue Size"="Img Save Que Size") -> (w252:T4)
            n147 = property on="Save buffer" class="WFChart (strict)"("YScale.Maximum"="Img Save Que Size") -> ()  [unwired: 2 in, 2 out]
          }
          event "Overload threshold": Value Change {
            w255 = State."Wait for Event"  # Next State
            # "Overload threshold (Image Processing)\nSet buffer size limit to overloading threshold. Values over this\nthreshold (while no object currently detected), will pause image\ncapture until image processing queue is empty."
            n148 = event-data() -> ()  [unwired: 1 in, 3 out]
            n149 = Bundle By Name(cluster=w256, "Overload threshold"="Overload threshold") -> (w257:T4)
          }
          event "Dispense Duration": Value Change {
            w260 = State."Wait for Event"  # Next State
            # "Dispense Duration (Pump speed)\nDescription..."
            n150 = event-data() -> ()  [unwired: 1 in, 3 out]
            n151 = Bundle By Name(cluster=w261, "Dispense Speed"="Dispense Duration") -> (w262:T4)
          }
          event "Flush Size": Value Change {
            w265 = State."Wait for Event"  # Next State
            # "Flush Size (Extra flush)\nDescription..."
            n152 = event-data() -> ()  [unwired: 1 in, 3 out]
            n153 = Bundle By Name(cluster=w266, "Flush Size"="Flush Size") -> (w267:T4)
          }
          event "Max Framerate": Value Change {
            w277 = State."Wait for Event"  # Next State
            # "Maximum Framerate\nMaximum image capture framerate."
            n154 = event-data() -> ()  [unwired: 1 in, 3 out]
            n155 = Unbundle By Name(w270) -> ("Exposure Time"=w275:dbl)
            n156 = Multiply(x=w275, y=10.0) -> (x*y=w274:dbl)
            n157 = Divide(x=1000000.0, y=w274) -> (x/y=w276:dbl)
            n158 = Max & Min(x="Max Framerate", y=w276) -> (min(x,y)=w269:dbl)  [unwired: 1 out]
            n159 = Bundle By Name(cluster=w270, "Max Framerate"="Max Framerate", "Framerate"=w269) -> (w278:T4)
            n160 = local write "Target framerate"(w269) -> ()
          }
          event "Light intensity": Value Change {
            # "Light Intensity\nChanges light intensity, value is  saved in \nsample information file."
            n161 = event-data() -> ()  [unwired: 1 in, 3 out]
            n162 = Bundle By Name(cluster=w283, "Light intensity"="Light intensity") -> (w282:T4)
          }
          event "New Sample timeout": Value Change {
            w286 = State."Wait for Event"  # Next State
            # "Sample Timeout\nDefined the timeout duration used to determine a new sample."
            n163 = event-data() -> ()  [unwired: 1 in, 3 out]
            n164 = Bundle By Name(cluster=w288, "Timeout Sample"="New Sample timeout") -> (w287:T4)
          }
          event "Sample size threshold": Value Change {
            w291 = State."Wait for Event"  # Next State
            # "Framerate\nDefined the save frequency (saves every nth image)\nValue saved in sample information file."
            n165 = event-data() -> ()  [unwired: 1 in, 3 out]
            n166 = Bundle By Name(cluster=w293, "Sample size threshold"="Sample size threshold") -> (w292:T4)
          }
          event "Max large object threshold": Value Change {
            # "Array size threshold\nChanges array size threshold, used to check if too many,\nobjects currently detected."
            n167 = event-data() -> ()  [unwired: 1 in, 3 out]
            n168 = Bundle By Name(cluster=w298, "Max large object threshold"="Max large object threshold") -> (w297:T4)
          }
          event "DetectCrop": Value Change {
            # "Movement Detection Crop %\nChanges the percentage of the image used for detecting\nmovement, before full image is tracked."
            n169 = event-data() -> ()  [unwired: 1 in, 3 out]
            n170 = Bundle By Name(cluster=w303, "Detection Region %"="DetectCrop") -> (w302:T4)
          }
          event "Change Crop": Value Change {
            w308 = State."Wait for Event"  # Next State
            # "Change crop\nChange the cropping of images."
            n171 = event-data() -> ()  [unwired: 1 in, 1 out]
            n172 = call "Camera_Crop_Setup.vi"("value"=w306) -> ("output cluster"=w305:T4)  [unwired: 10 in]
          }
        }
      }
      frame "Start Image Capture" {
        # "Start Image Capture\nActivating Camera and Image saving loops."
        n173 = call "Calibration_Load.vi"("Data in"=w312) -> ("Next State"=w311:T7, "Calibration error?"=w309:bool, "Data out"=w310:T4)  [unwired: 8 in]
        n174 = case shown="False" w309 {
          tunnel: [w319 w321] -> w313
          tunnel: w310 -> [w316 w321]
          frame False {
            # "Calibration image\nloaded succesfully."
            n175 = call "Capture_Save_Initialize.vi"("input cluster"=w316) -> ("output cluster"=w319:T4)  [unwired: 10 in]
            n176 = property on="Stop Image Capture" class="Bool"("DisabledEnum"=T8."Enabled" ("Disabled")) -> ()  [unwired: 2 in, 2 out]
            n177 = property on="Start Image Capture" class="Bool"("DisabledEnum"=T8."Disabled and Grayed Out" ("Disabled")) -> ()  [unwired: 2 in, 2 out]
            n178 = property on="Calibration Pictures" class="Bool"("DisabledEnum"=T8."Disabled and Grayed Out" ("Disabled")) -> ()  [unwired: 2 in, 2 out]
            "Active" <- TRUE ("Image_Capture")
          }
          frame True {
            # "Error loading calibration."
          }
        }
      }
      frame "Stop Image Capture" {
        w323 = T8."Enabled" ("Disabled")
        w326 = FALSE ("Image_Capture")
        w329 = State."Wait for Event"  # Next State
        # "Stop Image Capture\nStopping Camera and Image saving loops."
        n179 = call "Image_Acquisition_Stop.vi"("input cluster"=w325) -> ("output cluster"=w322:T4)  [unwired: 10 in]
        n180 = Bundle By Name(cluster=w322, "Img_Capt"=w326) -> (w327:T4)
        n181 = local write "Active"(w326) -> ()
        n182 = property on="Start Image Capture" class="Bool"("DisabledEnum"=w323) -> ()  [unwired: 2 in, 2 out]
        n183 = property on="Calibration Pictures" class="Bool"("DisabledEnum"=w323) -> ()  [unwired: 2 in, 2 out]
        n184 = property on="Stop Image Capture" class="Bool"("DisabledEnum"=T8."Disabled and Grayed Out" ("Disabled")) -> ()  [unwired: 2 in, 2 out]
      }
      frame "Calibration Pictures" {
        w330 = TRUE ("Crop?")
        # "Start Image Capture\nTake two calibration pictures with each camera and save in calibration folder."
        n185 = call "Calibration_Capture.vi"("Crop?"=FALSE, "value"=w340) -> ("Image2"=w336:T3, "Image1"=w337:T3, "output cluster"=w344:T4)  [unwired: 7 in]
        n186 = Unbundle By Name(w340) -> ("Img_Capt Begin"=w341:bool)
        n187 = local write "Camera 2 Detect"(w336) -> ()
        n188 = local write "Camera 1 Detect"(w337) -> ()
        n189 = call "Calibration_Capture.vi"("Detect Movement"=FALSE, "Crop?"=TRUE, "value"=w344) -> ("Image2"=w335:T3, "Image1"=w331:T3, "output cluster"=w332:T4)  [unwired: 6 in]
        n190 = local write "Camera 2 Binary"(w335) -> ()
        n191 = local write "Camera 1 Binary"(w331) -> ()
        n192 = call "Calibration_Capture.vi"("Detect Movement"=w330, "Crop?"=w330, "value"=w332) -> ("Image2"=w342:T3, "Image1"=w343:T3, "output cluster"=w338:T4)  [unwired: 6 in]
        n193 = case shown="False" w341 {
          tunnel: [w349 w353] -> w347
          tunnel: [w348 w351] -> w339
          tunnel: w338 -> [w348 w350]
          frame False {
            w349 = State."Wait for Event"  # Next State
          }
          frame True {
            w353 = State."Start Image Capture"  # Next State
            n194 = Bundle By Name(cluster=w350, "Img_Capt Begin"=FALSE) -> (w351:T4)
          }
        }
        n195 = local write "Camera 1"(w343) -> ()
        n196 = local write "Camera 2"(w342) -> ()
      }
      frame "Empty and Refill" {
        w368 = T8."Enabled" ("Disabled")
        w366 = TRUE ("Empty_Refill")
        w372 = FALSE ("Image_Capture")
        w376 = State."Valve Signal"  # Next State
        # "Load extra flush volume"
        # "Empty and Refill command\nActivate Empty and refill of cuvette, start listening for valve return signal."
        n197 = Unbundle By Name(w370) -> ("XE 1000 Pump"=w361:refnum<visa-resource-name>, "L16 Linear Actuator"=w373:refnum<visa-resource-name>, "Flush Size"=w354:i32)
        n198 = Number To Decimal String(number=w354) -> (decimal integer string=w357:string)  [unwired: 1 in]
        n199 = Greater Than 0?(x=w354) -> (x > 0?=w355:bool)
        n200 = Concatenate Strings("/1IS20A" ("write buffer 2"), w357, "R" ("string"), "\r\n") -> (w363:string)
        n201 = property on="Empty and Refill" class="Bool"("DisabledEnum"=T8."Disabled and Grayed Out" ("Disabled")) -> ()  [unwired: 2 in, 2 out]
        n202 = property on="Stop Image Capture" class="Bool"("DisabledEnum"=T8."Disabled and Grayed Out" ("Disabled")) -> ()  [unwired: 2 in, 2 out]
        n203 = property on="Start Image Capture" class="Bool"("DisabledEnum"=w368) -> ()  [unwired: 2 in, 2 out]
        n204 = property on="Calibration Pictures" class="Bool"("DisabledEnum"=w368) -> ()  [unwired: 2 in, 2 out]
        n205 = VISA Write(VISA resource name=w373, write buffer="102", error in (no error)=w365) -> (error out=w360:errorcluster)  [unwired: 2 out]
        n206 = case shown="False" w355 {
          tunnel: w363 -> [_ w381]
          tunnel: w361 -> [_ w380]
          tunnel: w360 -> [w377 w379]
          tunnel: [w377 w378] -> w359
          frame False {
          }
          frame True {
            n207 = VISA Write(VISA resource name=w380, write buffer=w381, error in (no error)=w379) -> (error out=w378:errorcluster)  [unwired: 2 out]
          }
        }
        n208 = call "Image_Acquisition_Stop.vi"("input cluster"=w370) -> ("output cluster"=w364:T4)  [unwired: 10 in]
        n209 = Tick Count (ms)() -> (millisecond timer value=w367:u32)
        n210 = Bundle By Name(cluster=w364, "Img_Capt"=w372, "Empty_Refill"=w366, "Open(T)/Close(F)"=w366, "Empty start"=w367) -> (w375:T4)
        n211 = local write "Active"(w372) -> ()
      }
      frame "Close and Refill" {
        w393 = T8."Enabled" ("Disabled")
        w397 = FALSE ("Image_Capture")
        w401 = State."Valve Signal"  # Next State
        # "Empty and Refill command\nActivate Empty and refill of cuvette, start listening for valve return signal."
        n212 = Unbundle By Name(w395) -> ("XE 1000 Pump"=w385:refnum<visa-resource-name>, "L16 Linear Actuator"=w398:refnum<visa-resource-name>)
        n213 = VISA Write(VISA resource name=w398, write buffer="101", error in (no error)=w390) -> (error out=w384:errorcluster)  [unwired: 2 out]
        n214 = Concatenate Strings("/1IS20A810R" ("write buffer 2"), "\r\n") -> (w388:string)
        n215 = property on="Empty and Refill" class="Bool"("DisabledEnum"=T8."Disabled and Grayed Out" ("Disabled")) -> ()  [unwired: 2 in, 2 out]
        n216 = property on="Stop Image Capture" class="Bool"("DisabledEnum"=T8."Disabled and Grayed Out" ("Disabled")) -> ()  [unwired: 2 in, 2 out]
        n217 = property on="Start Image Capture" class="Bool"("DisabledEnum"=w393) -> ()  [unwired: 2 in, 2 out]
        n218 = property on="Calibration Pictures" class="Bool"("DisabledEnum"=w393) -> ()  [unwired: 2 in, 2 out]
        n219 = VISA Write(VISA resource name=w385, write buffer=w388, error in (no error)=w384) -> (error out=w383:errorcluster)  [unwired: 2 out]
        n220 = call "Image_Acquisition_Stop.vi"("input cluster"=w395) -> ("output cluster"=w389:T4)  [unwired: 10 in]
        n221 = Tick Count (ms)() -> (millisecond timer value=w392:u32)
        n222 = Bundle By Name(cluster=w389, "Img_Capt"=w397, "Empty_Refill"=TRUE, "Open(T)/Close(F)"=FALSE, "Empty start"=w392) -> (w400:T4)
        n223 = local write "Active"(w397) -> ()
      }
      frame "Valve Signal" {
        # "Listen for valve return signal\nListen for valve return signal indicating valve is OPEN or CLOSED."
        n224 = call "Empty_Complete.vi"("input cluster"=w411) -> ("Next State"=w407:T7, "output cluster"=w402:T4)  [unwired: 9 in]
        n225 = local read "Pump"() -> (w403:bool)
        n226 = Equal?(x=State."Pump Cycle" ("Next State"), y=w407) -> (x = y?=w406:bool)
        n227 = Equal?(x=w407, y=State."Wait for Event" ("Next State")) -> (x = y?=w405:bool)
        n228 = Or(x=w406, y=w405) -> (x .or. y?=w404:bool)
        n229 = case shown="True" w404 {
          tunnel: w403 -> [_ w413]
          frame False {
          }
          frame True {
            w412 = T8."Enabled" ("Disabled")
            n230 = case shown="True" w413 {
              frame False {
              }
              frame True {
                n231 = property on="Empty and Refill" class="Bool"("DisabledEnum"=T8."Enabled" ("Disabled")) -> ()  [unwired: 2 in, 2 out]
              }
            }
            n232 = property on="Start Image Capture" class="Bool"("DisabledEnum"=w412) -> ()  [unwired: 2 in, 2 out]
            n233 = property on="Empty Cuvette" class="Bool"("DisabledEnum"=w412) -> ()  [unwired: 2 in, 2 out]
            n234 = property on="Calibration Pictures" class="Bool"("DisabledEnum"=w412) -> ()  [unwired: 2 in, 2 out]
          }
        }
      }
      frame "Position" {
        w424 = State."Wait for Event"  # Next State
        # "Read linear actuator position\nSend command and read linear actuator position."
        n235 = Unbundle By Name(w428) -> ("L16 Linear Actuator"=w427:refnum<visa-resource-name>)
        n236 = VISA Write(VISA resource name=w427, write buffer="104", error in (no error)=w425) -> (VISA resource name out=w417:refnum<visa-resource-name>, error out=w423:errorcluster)  [unwired: 1 out]
        n237 = call "Stall Data Flow.vim"("value in"=w417, "milliseconds to wait"=u32 500) -> ("value out"=w415:refnum<visa-resource-name>)  [unwired: 1 out]
        n238 = property class="Instr"(reference=w415, error in=w423) -> (reference out=w421:refnum<visa-resource-name>, error out=w420:errorcluster, "Serial Settings:Number of Bytes at Serial Port"=w422:u32)
        n239 = VISA Read(VISA resource name=w421, byte count=w422, error in (no error)=w420) -> (read buffer=→"Current Position":string, error out=w418:errorcluster)  [unwired: 2 out]
      }
      frame "Valve Cycle" {
        w432 = T8."Enabled" ("Disabled")
        w431 = T8."Disabled and Grayed Out" ("Disabled")
        w435 = FALSE ("Image_Capture")
        w441 = State."Valve Signal"  # Next State
        # "Manual cycle of linear actuator\nRetract and extend linear actuator."
        n240 = Unbundle By Name(w433) -> ("L16 Linear Actuator"=w440:refnum<visa-resource-name>)
        n241 = VISA Write(VISA resource name=w440, write buffer="102", error in (no error)=w439) -> (error out=w438:errorcluster)  [unwired: 2 out]
        n242 = property on="Start Image Capture" class="Bool"("DisabledEnum"=w432) -> ()  [unwired: 2 in, 2 out]
        n243 = property on="Calibration Pictures" class="Bool"("DisabledEnum"=w432) -> ()  [unwired: 2 in, 2 out]
        n244 = property on="Stop Image Capture" class="Bool"("DisabledEnum"=w431) -> ()  [unwired: 2 in, 2 out]
        n245 = property on="Empty Cuvette" class="Bool"("DisabledEnum"=w431) -> ()  [unwired: 2 in, 2 out]
        n246 = call "Image_Acquisition_Stop.vi"("input cluster"=w433) -> ("output cluster"=w430:T4)  [unwired: 10 in]
        n247 = Tick Count (ms)() -> (millisecond timer value=w436:u32)
        n248 = Bundle By Name(cluster=w430, "Open(T)/Close(F)"=TRUE, "Img_Capt"=w435, "Empty_Refill"=w435, "Empty start"=w436) -> (w434:T4)
      }
      frame "Valve Open" {
        w449 = State."Wait for Event"  # Next State
        w443 = T8."Disabled and Grayed Out" ("Disabled")
        # "Manual extend of linear actuator\nSend extend command to linear actuator."
        n249 = Unbundle By Name(w447) -> ("L16 Linear Actuator"=w451:refnum<visa-resource-name>)
        n250 = VISA Write(VISA resource name=w451, write buffer="102", error in (no error)=w452) -> (error out=w450:errorcluster)  [unwired: 2 out]
        n251 = property on="Calibration Pictures" class="Bool"("DisabledEnum"=w443) -> ()  [unwired: 2 in, 2 out]
        n252 = property on="Start Image Capture" class="Bool"("DisabledEnum"=w443) -> ()  [unwired: 2 in, 2 out]
        n253 = property on="Stop Image Capture" class="Bool"("DisabledEnum"=w443) -> ()  [unwired: 2 in, 2 out]
        n254 = call "Image_Acquisition_Stop.vi"("input cluster"=w447) -> ("output cluster"=w445:T4)  [unwired: 10 in]
        n255 = Bundle By Name(cluster=w445, "Img_Capt"=FALSE ("Image_Capture"), "Open(T)/Close(F)"=TRUE) -> (w444:T4)
      }
      frame "Valve Close" {
        w462 = State."Valve Signal"  # Next State
        # "Manual retract of linear actuator\nSend retract command to linear actuator."
        n256 = Unbundle By Name(w460) -> ("Empty_Refill"=w456:bool, "XE 1000 Pump"=w454:refnum<visa-resource-name>, "L16 Linear Actuator"=w463:refnum<visa-resource-name>)
        n257 = VISA Write(VISA resource name=w463, write buffer="101", error in (no error)=w464) -> (error out=w455:errorcluster)  [unwired: 2 out]
        n258 = case shown="True" w456 {
          tunnel: w455 -> [w465 w471]
          tunnel: w454 -> [_ w470]
          tunnel: [w465 w466] -> w453
          frame False {
            # "Manual Close, don't load volume."
          }
          frame True {
            # "Load specified volume in pump."
            n259 = Concatenate Strings("/1IS20A810R" ("write buffer 2"), "\r\n") -> (w467:string)
            n260 = VISA Write(VISA resource name=w470, write buffer=w467, error in (no error)=w471) -> (error out=w466:errorcluster)  [unwired: 2 out]
          }
        }
        n261 = Tick Count (ms)() -> (millisecond timer value=w458:u32)
        n262 = Bundle By Name(cluster=w460, "Empty start"=w458, "Open(T)/Close(F)"=FALSE) -> (w459:T4)
      }
      frame "Pump Command" {
        w480 = State."Wait for Event"  # Next State
        # "<I> Input valve\n<A> Absolute position (n = 1...1000)\n<O> Output valve\n<R> Execute commands\n<T> Abort commands"
        # "Pump command\nSend command to XE 1000 Pump."
        n263 = Unbundle By Name(w479) -> ("XE 1000 Pump"=w476:refnum<visa-resource-name>, "Command"=w473:string)
        n264 = Concatenate Strings("/1" ("string"), w473, "\r\n") -> (w477:string)
        n265 = VISA Write(VISA resource name=w476, write buffer=w477, error in (no error)=w475) -> (error out=w474:errorcluster)  [unwired: 2 out]
      }
      frame "Pump Cycle" {
        w490 = State."Wait for Event"  # Next State
        # "<I> Input valve\n<A> Absolute position (n = 1...1000)\n<O> Output valve\n<R> Execute commands\n<T> Abort commands"
        # "Pump Cycle\nSend command to XE 1000 Pump going through full cycle."
        n266 = Unbundle By Name(w484) -> ("Empty_Refill"=w489:bool, "XE 1000 Pump"=w488:refnum<visa-resource-name>, "Dispense Speed"=w482:i32)
        n267 = Number To Decimal String(number=w482) -> (decimal integer string=w481:string)  [unwired: 1 in]
        n268 = case shown="False" w489 {
          tunnel: w488 -> [w502 w512]
          tunnel: w487 -> [w499 w509]
          tunnel: [w498 w508] -> w486
          tunnel: [u32 3000 ("milliseconds to wait") u32 5000 ("milliseconds to wait")] -> w485
          tunnel: w484 -> [w495 w506]
          tunnel: [w494 w506] -> w483
          tunnel: w481 -> [w492 w504]
          frame True {
            # "Dispense ready volume."
            n269 = Concatenate Strings("/1S" ("write buffer 2"), w492, "OA0R" ("string"), "\r\n") -> (w500:string)
            n270 = Bundle By Name(cluster=w495, "Empty_Refill"=FALSE) -> (w494:T4)
            n271 = VISA Write(VISA resource name=w502, write buffer=w500, error in (no error)=w499) -> (error out=w498:errorcluster)  [unwired: 2 out]
          }
          frame False {
            # "Load and dispense volume."
            n272 = Concatenate Strings("/1IS20A810S" ("write buffer 2"), w504, "OA0R" ("string"), "\r\n") -> (w510:string)
            n273 = VISA Write(VISA resource name=w512, write buffer=w510, error in (no error)=w509) -> (error out=w508:errorcluster)  [unwired: 2 out]
          }
        }
        n274 = Wait (ms)(milliseconds to wait=w485) -> ()  [unwired: 1 out]
      }
      frame "Extra Flush" {
        w520 = State."Valve Close"  # Next State
        # "<I> Input valve\n<A> Absolute position (n = 1...1000)\n<O> Output valve\n<R> Execute commands\n<T> Abort commands"
        # "Pump Extra Flush\nSend command to XE 1000 Pump dispensing an extra flush to clean Cuvette"
        n275 = Unbundle By Name(w519) -> ("XE 1000 Pump"=w515:refnum<visa-resource-name>, "Dispense Speed"=w517:i32)
        n276 = Greater Than 0?(x=w517) -> (x > 0?=w518:bool)
        n277 = Number To Decimal String(number=w517) -> (decimal integer string=w514:string)  [unwired: 1 in]
        n278 = case shown="True" w518 {
          tunnel: w516 -> [w521 w528]
          tunnel: w515 -> [_ w527]
          tunnel: w514 -> [_ w525]
          tunnel: [w521 w522] -> w513
          frame False {
          }
          frame True {
            n279 = Concatenate Strings("/1S" ("write buffer 2"), w525, "OA0R" ("string"), "\r\n") -> (w529:string)
            n280 = VISA Write(VISA resource name=w527, write buffer=w529, error in (no error)=w528) -> (error out=w522:errorcluster)  [unwired: 2 out]
            n281 = Wait (ms)(milliseconds to wait=u32 2000) -> ()  [unwired: 1 out]
          }
        }
      }
      frame "Start System" {
        w542 = State."Empty and Refill"  # Next State
        # "Y<n>: Initialize (Right input, Left output)  (<n> = speed 2-20 sec/stroke)\nS:<n>: Set speed (<n> = 20..600 strokes in 1/10 sec).\nA<n>: Absolute position (<n> = 1...1000)\nI: Input valve\nO: Output valve\nR: Execute commands\nT: Abort commands"
        # "Pump Initialize\nInitialize XE 1000 Pump and fill tubes, emptying cuvette and refill to full."
        n282 = Unbundle By Name(w532) -> ("XE 1000 Pump"=w540:refnum<visa-resource-name>)
        n283 = Concatenate Strings("/1Y5IS20A810S60OA0R" ("string"), "\r\n") -> (w541:string)
        n284 = VISA Write(VISA resource name=w540, write buffer=w541, error in (no error)=w539) -> (error out=w538:errorcluster)  [unwired: 2 out]
        n285 = Wait (ms)(milliseconds to wait=u32 10000) -> ()  [unwired: 1 out]
        n286 = property on="Empty and Refill" class="Bool"("DisabledEnum"=T8."Enabled" ("Disabled")) -> ()  [unwired: 2 in, 2 out]
        n287 = Bundle By Name(cluster=w532, "Img_Capt"=FALSE) -> (w531:T4)
      }
      frame "Empty System" {
        w560 = State."Valve Cycle"  # Next State
        # "<I> Input valve\n<A> Absolute position (n = 1...1000)\n<O> Output valve\n<R> Execute commands\n<T> Abort commands"
        # "Empty pump and pipes\nSend command to XE 1000 Pump and empty system."
        n288 = Unbundle By Name(w544) -> ("XE 1000 Pump"=w558:refnum<visa-resource-name>)
        n289 = Concatenate Strings("/1OS20A1000IA0" ("write buffer 2"), "OS20A1000IA0" ("write buffer 2"), "R" ("write buffer 2")) -> (w553:string)
        n290 = Concatenate Strings(w553, "\r\n") -> (w547:string)
        n291 = VISA Write(VISA resource name=w558, write buffer=w547, error in (no error)=w557) -> (VISA resource name out=w552:refnum<visa-resource-name>, error out=w549:errorcluster)  [unwired: 1 out]
        n292 = property on="Empty and Refill" class="Bool"("DisabledEnum"=T8."Disabled and Grayed Out" ("Disabled")) -> ()  [unwired: 2 in, 2 out]
        n293 = call "Stall Data Flow.vim"("value in"=w552, "milliseconds to wait"=u32 10000) -> ("value out"=w551:refnum<visa-resource-name>)  [unwired: 1 out]
        n294 = VISA Write(VISA resource name=w551, write buffer=w547, error in (no error)=w549) -> (error out=w548:errorcluster)  [unwired: 2 out]
        n295 = Bundle By Name(cluster=w544, "Img_Capt"=FALSE) -> (w543:T4)
      }
      frame "Change Light Intensity" {
        w563 = State."Wait for Event"  # Next State
        # "Manual extend of linear actuator\nSend extend command to linear actuator."
        n296 = Unbundle By Name(w567) -> ("L16 Linear Actuator"=w565:refnum<visa-resource-name>, "Light intensity"=w562:i32)
        n297 = Number To Decimal String(number=w562) -> (decimal integer string=w561:string)  [unwired: 1 in]
        n298 = VISA Write(VISA resource name=w565, write buffer=w561, error in (no error)=w566) -> (error out=w564:errorcluster)  [unwired: 2 out]
      }
      frame "Exit" {
        w571 = FALSE ("Pump")
        w573 = FALSE ("Pump")
        w575 = TRUE  # Stop Loop?
        w576 = State."Exit"  # (Value Not Used)
        # "Exit application\nClose all connections, destroy memory allocations, and Exit the application. \n(Potential for saving a settings file)"
        n299 = call "Terminate_Connection.vi"("error in"=w574, "Data"=w569) -> ("error out"=w570:errorcluster)  [unwired: 8 in, 1 out]
        n300 = call "Settings_Save.vi"("error in"=w570, "input cluster"=w569) -> ("error out"=w568:errorcluster)  [unwired: 9 in]
        n301 = local write "Active"(w573) -> ()
        n302 = local write "Camear 1"(w573) -> ()
        n303 = local write "Camera 2"(w573) -> ()
        n304 = local write "Pump"(w573) -> ()
        n305 = local write "Actuator"(w573) -> ()
        n306 = Bundle By Name(cluster=w569, "Img_Capt"=w571, "Actuator"=w571, "Pump"=w571, "Cam 1"=w571, "Cam 2"=w571) -> (w572:T4)
      }
    }
    n307 = Or(x=w12, y=FALSE) -> (x .or. y?=w14:bool)
    n308 = call <extravilib>:"Write.vi"("element"=w16) -> ("channel"=w11:T10)  [unwired: 1 out]
    n309 = call <extravilib>:"Write.vi"("element"=w14) -> ("channel"=w10:T11)  [unwired: 1 out]
  }
  n310 = call <vilib>:"Simple Error Handler.vi"("error in (no error)"=w6) -> ("error out"=w5:errorcluster)  [unwired: 4 in, 4 out]
  n311 = disable-structure shown="RUN_TIME_ENGINE==True" {
    disable-tunnel: w5 -> [_ _]
    frame condition #0 (active) {
    }
    frame condition #1 {
      # "Call Quit LabVIEW if running as a built application."
      n312 = Quit LabVIEW() -> ()  [unwired: 1 in]
    }
  }
  n313 = while {
    tunnel: w3 -> [w578]
    tunnel: w2 -> [w582]
    tunnel: [w577] -> w1
    stop <- w584 stop-if-true
    # "Image handling - object detection"
    n314 = call <extravilib>:"Read.vi"("channel"=w582) -> ("element"=w580:T4)  [unwired: 1 in, 1 out]
    n315 = Unbundle By Name(w580) -> ("Img_Capt"=w581:bool)
    n316 = case shown="True" w581 {
      tunnel: [TRUE ("Last Image?") w593] -> w583
      tunnel: w582 -> [_ w594]
      tunnel: [w587 w592] -> w577
      frame False {
        # "Image capture inactive"
        n317 = Bundle(TRUE, FALSE) -> (w588:cluster{bool, bool})  [unwired: 1 in]
        n318 = call <extravilib>:"Write.vi"("element"=w588) -> ("channel"=w587:T12)  [unwired: 1 out]
        n319 = local write "Process buffer"(T2 {"# elements in queue"=0, "# elements in queue"=0} ("Image processing")) -> ()
        n320 = Wait (ms)(milliseconds to wait=u32 10) -> ()  [unwired: 1 out]
      }
      frame True {
        # "Image capture active"
        n321 = while "Save image" {
          tunnel: w594 -> [w600]
          tunnel: [w601] -> w593
          tunnel: [w595] -> w592
          stop <- w601 stop-if-true
          # "Image Processing"
          n322 = call <extravilib>:"Read.vi"("channel"=w600) -> ("element"=w599:T4)  [unwired: 1 in, 1 out]
          n323 = call "Image_Processing_Queue.vi"("Data"=w599) -> ("Status"=w595:T12, "Process queue"=→"Process buffer":T2, "Last Image?"=w601:bool, "Image 1"=→"Camera 1":T3, "Image 2"=→"Camera 2":T3, "Binary 1"=→"Camera 1 Binary":T3, "Binary 2"=→"Camera 2 Binary":T3)  [unwired: 10 in, 2 out]
        }
      }
    }
    n324 = call <extravilib>:"Read.vi"("channel"=w578) -> ("element"=w579:bool)  [unwired: 1 in, 1 out]
    n325 = And(x=w583, y=w579) -> (x .and. y?=w584:bool)
  }
  n326 = while {
    tunnel: w3 -> [w614]
    tunnel: w2 -> [w613]
    tunnel: w1 -> [w607]
    stop <- w611 stop-if-true
    # "Camera Handler"
    n327 = call <extravilib>:"Read.vi"("channel"=w607) -> ("element"=w606:cluster{bool, bool})  [unwired: 1 in, 1 out]
    n328 = call <extravilib>:"Read.vi"("channel"=w613) -> ("element"=w612:T4)  [unwired: 1 in, 1 out]
    n329 = Unbundle(w606) -> (w604:bool, w605:bool)
    n330 = Unbundle By Name(w612) -> ("Img_Capt"=w609:bool)
    n331 = call <extravilib>:"Read.vi"("channel"=w614) -> ("element"=w611:bool)  [unwired: 1 in, 1 out]
    n332 = Not(x=w605) -> (.not. x?=w610:bool)
    n333 = And(x=w610, y=w609) -> (x .and. y?=w608:bool)
    n334 = case shown="True" w608 {
      tunnel: w612 -> [_ w618]
      tunnel: w604 -> [_ w617]
      frame False {
        # "Empty Case\nImage Capture currently inactive."
        n335 = local write "Framerate"(0.0 ("Framerate")) -> ()
        n336 = Wait (ms)(milliseconds to wait=u32 20) -> ()  [unwired: 1 out]
      }
      frame True {
        # "Capture Image\nImage Capture currently active, transmitting data."
        n337 = call "Image_Snap_Dual.vi"("input cluster"=w618, "Detect Movement"=w617) -> ("Framerate"=→"Framerate":i32)  [unwired: 6 in, 3 out]
      }
    }
  }
  n338 = while {
    tunnel: w2 -> [w624]
    tunnel: w3 -> [w622]
    tunnel: w2 -> [w620]
    stop <- w626 stop-if-true
    # "Image Save"
    n339 = call <extravilib>:"Read.vi"("channel"=w624) -> ("element"=w623:T4)  [unwired: 1 in, 1 out]
    n340 = call <extravilib>:"Read.vi"("channel"=w622) -> ("element"=w625:bool)  [unwired: 1 in, 1 out]
    n341 = Unbundle By Name(w623) -> ("Img_Capt"=w627:bool)
    n342 = case shown="True" w627 {
      selector: w627 -> [_ w632]
      tunnel: w622 -> [_ w635]
      tunnel: [TRUE ("Last Image?") w633] -> w621
      tunnel: w620 -> [_ w634]
      frame False {
        n343 = local write "Save buffer"(T2 {"# elements in queue"=0, "# elements in queue"=0} ("Image Saving")) -> ()
        n344 = Wait (ms)(milliseconds to wait=u32 10) -> ()  [unwired: 1 out]
      }
      frame True {
        n345 = while {
          tunnel: w635 -> [w646]
          tunnel: w634 -> [w645]
          tunnel: [w642] -> w633
          shift-right: [FALSE] -> _
          shift-left: w632 -> [w638]
          stop <- w642 stop-if-true
          n346 = call <extravilib>:"Read.vi"("channel"=w645) -> ("element"=w644:T4)  [unwired: 1 in, 1 out]
          n347 = call <extravilib>:"Read.vi"("channel"=w646) -> ("element"=w643:bool)  [unwired: 1 in, 1 out]
          n348 = call "Image_Save_Handler.vi"("Stop?"=w643, "Data"=w644, "first iteration"=w638) -> ("Stop out"=w642:bool, "timeout"=→"Ready":bool, "Queue size"=→"Save buffer":T2, "Image Save 2"=→"Camera 2 Detect":T3, "Image Save 1"=→"Camera 1 Detect":T3)  [unwired: 3 in, 1 out]
        }
      }
    }
    n349 = And(x=w621, y=w625) -> (x .and. y?=w626:bool)
    n350 = case shown="True" w626 {
      frame False {
      }
      frame True {
        n351 = call "IMAQ Dispose"("All Images? (No)"=TRUE) -> ()  [unwired: 5 in, 1 out]
      }
    }
  }
